vi "Create Cursor Object.vi"(4 "Cursor ID":i32, 5 "Cursor Property":T1, 7 "Range Property":T11, 8 "error in (no error)":errorcluster, 9 "Actual Transform In":T9, 11 "Cursor Object In":refnum<vi>) -> (0 "error out":errorcluster, 1 "Actual Transform Out":T9, 3 "Cursor Object Out":refnum<vi>)   [LabVIEW 2020, in "3D Plot.lvclass"]
uses:
  3D Plot.lvclass
  Range Property.ctl
  Range Clusters.ctl
  Actual Transform.ctl
  Cursor Property.ctl
  Cursor Position.ctl
  Cursor Point.ctl
  Sprite Type.ctl
  Cursor Line.ctl
  Line Type.ctl
  Cursor Plane.ctl
  Cursor Text.ctl
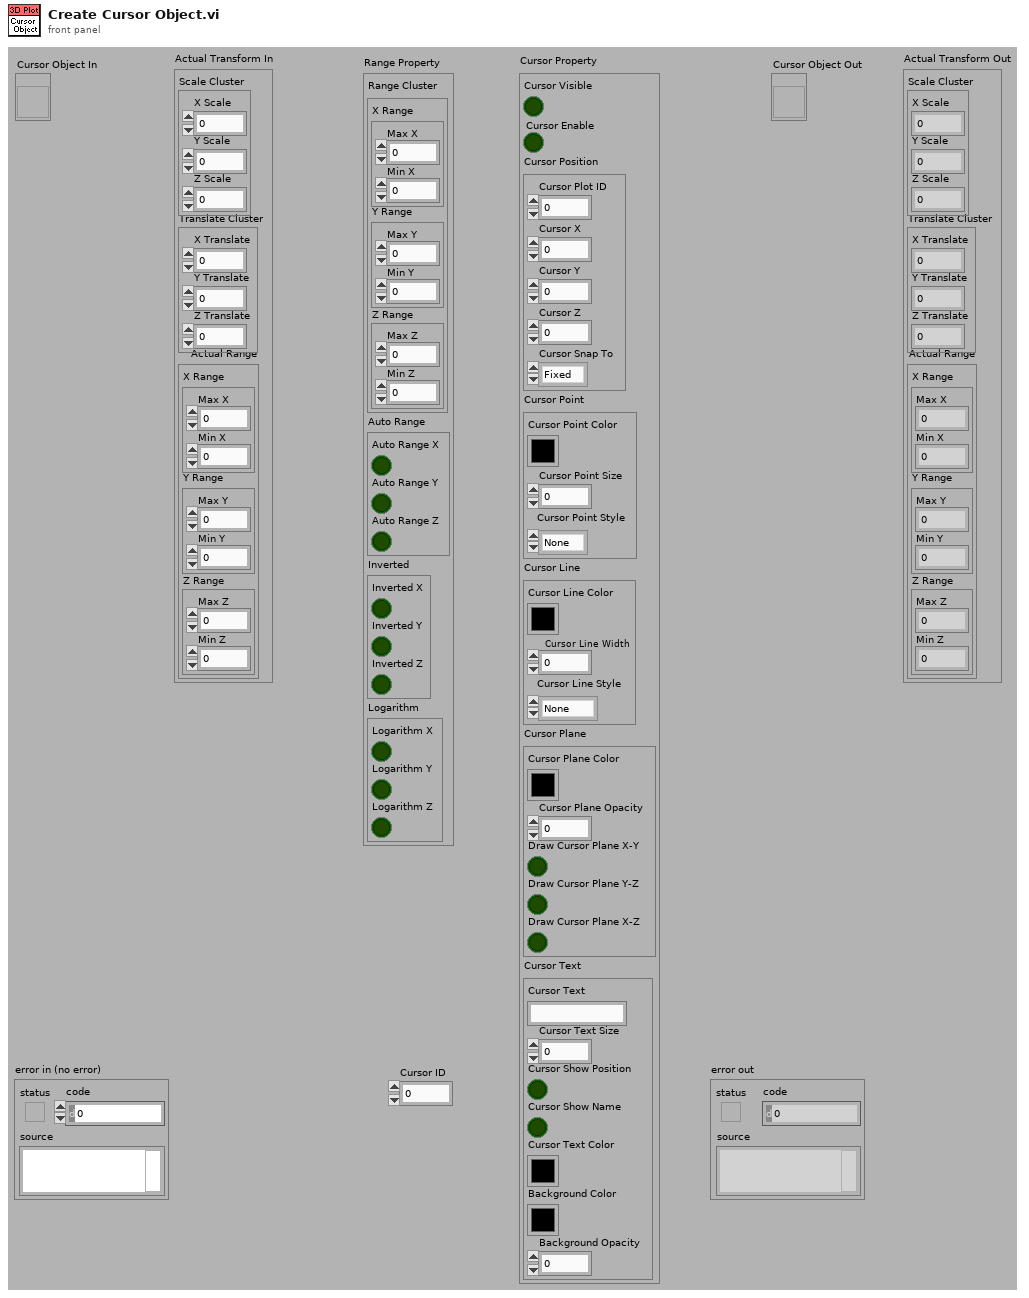
[diagram p1: front panel]
types:
  T1 = typedef "3D Plot.lvclass/Cursor Property.ctl" = cluster{"Cursor Visible":bool, "Cursor Enable":bool, "Cursor Position":T2, "Cursor Point":T3, "Cursor Line":T5, "Cursor Plane":T7, "Cursor Text":T8}
  T2 = typedef "3D Plot.lvclass/Cursor Position.ctl" = cluster{"Cursor Plot ID":i32, "Cursor X":sgl, "Cursor Y":sgl, "Cursor Z":sgl, "Cursor Snap To":enum16{"Fixed", "Nearest Plot", "Snap to Plot"}}
  T3 = typedef "3D Plot.lvclass/Cursor Point.ctl" = cluster{"Cursor Point Color":u32, "Cursor Point Size":sgl, "Cursor Point Style":T4}
  T4 = typedef "3D Plot.lvclass/Sprite Type.ctl" = enum16{"None", "Empty Square", "Solid Square", "Empty Diamond", "Solid Diamond", "Empty Circle", "Solid Circle", "Asterisk", "Bold X", "Wireframe Sphere", "Solid Sphere", "Wireframe Cube", "Solid Cube"}
  T5 = typedef "3D Plot.lvclass/Cursor Line.ctl" = cluster{"Cursor Line Color":u32, "Cursor Line Width":sgl, "Cursor Line Style":T6}
  T6 = typedef "3D Plot.lvclass/Line Type.ctl" = enum16{"None", "Solid", "Dash", "Dot", "Dash Dot"}
  T7 = typedef "3D Plot.lvclass/Cursor Plane.ctl" = cluster{"Cursor Plane Color":u32, "Cursor Plane Opacity":sgl, "Draw Cursor Plane X-Z":bool, "Draw Cursor Plane Y-Z":bool, "Draw Cursor Plane X-Y":bool}
  T8 = typedef "3D Plot.lvclass/Cursor Text.ctl" = cluster{"Cursor Text":string, "Cursor Text Size":u16, "Cursor Show Position":bool, "Cursor Show Name":bool, "Cursor Text Color":u32, "Background Color":u32, "Background Opacity":sgl}
  T9 = typedef "3D Plot.lvclass/Actual Transform.ctl" = cluster{"Scale Cluster":cluster{"X Scale":sgl, "Y Scale":sgl, "Z Scale":sgl}, "Translate Cluster":cluster{"X Translate":sgl, "Y Translate":sgl, "Z Translate":sgl}, "Actual Range":T10}
  T10 = typedef "3D Plot.lvclass/Range Clusters.ctl" = cluster{"X Range":cluster{"Max X":sgl, "Min X":sgl}, "Y Range":cluster{"Max Y":sgl, "Min Y":sgl}, "Z Range":cluster{"Max Z":sgl, "Min Z":sgl}}
  T11 = typedef "3D Plot.lvclass/Range Property.ctl" = cluster{"Range Cluster":T10, "Auto Range":cluster{"Auto Range X":bool, "Auto Range Y":bool, "Auto Range Z":bool}, "Inverted":cluster{"Inverted X":bool, "Inverted Y":bool, "Inverted Z":bool}, "Logarithm":cluster{"Logarithm X":bool, "Logarithm Y":bool, "Logarithm Z":bool}}
  T12 = cluster{"X Scale":sgl, "Y Scale":sgl, "Z Scale":sgl}
  T13 = cluster{"Cursor Value Out":sgl, "Cursor Value Out":sgl, "Cursor Value Out":sgl}
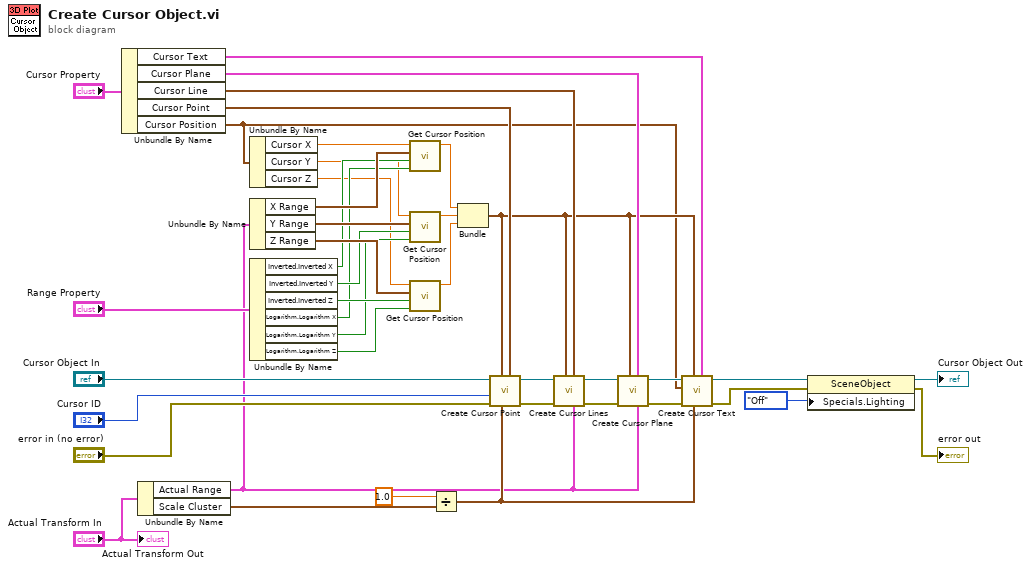
[diagram p0: block diagram]
diagram:
  n1 = Unbundle By Name("Cursor Property") -> ("Cursor Text"=w24:T8, "Cursor Plane"=w29:T7, "Cursor Line"=w32:T5, "Cursor Point"=w36:T3, "Cursor Position"=w1:T2)
  n2 = Unbundle By Name("Actual Transform In") -> ("Actual Range"=w9:T10, "Scale Cluster"=w39:T12)
  n3 = Unbundle By Name(w1) -> ("Cursor X"=w8:sgl, "Cursor Y"=w7:sgl, "Cursor Z"=w6:sgl)
  n4 = Unbundle By Name(w9) -> ("X Range"=w14:cluster{"Max X":sgl, "Min X":sgl}, "Y Range"=w15:cluster{"Max Y":sgl, "Min Y":sgl}, "Z Range"=w18:cluster{"Max Z":sgl, "Min Z":sgl})
  n5 = Unbundle By Name("Range Property") -> ("Inverted.Inverted X"=w12:bool, "Inverted.Inverted Y"=w16:bool, "Inverted.Inverted Z"=w19:bool, "Logarithm.Logarithm X"=w13:bool, "Logarithm.Logarithm Y"=w17:bool, "Logarithm.Logarithm Z"=w20:bool)
  n6 = call "Get Cursor Position.vi"("Logarithm?"=w13, "Inverted?"=w12, "Range"=w14, "Cursor Value In"=w8) -> ("Cursor Value Out"=w5:sgl)  [unwired: 7 out]
  n7 = call "Get Cursor Position.vi"("Logarithm?"=w17, "Inverted?"=w16, "Range"=w15, "Cursor Value In"=w7) -> ("Cursor Value Out"=w4:sgl)  [unwired: 7 out]
  n8 = call "Get Cursor Position.vi"("Logarithm?"=w20, "Inverted?"=w19, "Range"=w18, "Cursor Value In"=w6) -> ("Cursor Value Out"=w3:sgl)  [unwired: 7 out]
  n9 = Divide(x=sgl 1.0, y=w39) -> (x/y=w10:T12)
  n10 = Bundle("Cursor Value Out"=w5, "Cursor Value Out"=w4, "Cursor Value Out"=w3) -> (w2:T13)  [unwired: 1 in]
  n11 = call "Create Cursor Point.vi"("Cursor Point"=w36, "Scale"=w10, "Cursor Position"=w2, "error in (no error)"="error in (no error)", "Cursor ID"="Cursor ID", "Cursor Object In"="Cursor Object In") -> ("error out"=w33:errorcluster, "Cursor Object Out"=w34:refnum<vi>)  [unwired: 1 in, 3 out]
  n12 = call "Create Cursor Lines.vi"("Actual Range"=w9, "Cursor Line"=w32, "Cursor Position"=w2, "error in (no error)"=w33, "Cursor Object In"=w34) -> ("error out"=w30:errorcluster, "Cursor Object Out"=w31:refnum<vi>)  [unwired: 5 out]
  n13 = call "Create Cursor Plane.vi"("Actual Range"=w9, "Cursor Plane"=w29, "Cursor Position"=w2, "error in (no error)"=w30, "Cursor Object In"=w31) -> ("error out"=w27:errorcluster, "Cursor Object Out"=w28:refnum<vi>)  [unwired: 5 out]
  n14 = call "Create Cursor Text.vi"("Cursor Text"=w24, "Scale"=w10, "Cursor Position"=w2, "error in (no error)"=w27, "Cursor Property"=w1, "Cursor Object In"=w28) -> ("error out"=w26:errorcluster, "Cursor Object Out"=w25:refnum<vi>)  [unwired: 2 in, 2 out]
  n15 = property class="SceneObject"(reference=w25, error in=w26, "Specials.Lighting"=enum16{"Inherit Value", "Off", "On"}."Off" ("Specials:Lighting")) -> (reference out=→"Cursor Object Out":refnum<vi>, error out=→"error out":errorcluster)
  "Actual Transform Out" <- "Actual Transform In"
